vi "SN_parser_new.vi"(6 "Length range":T1, 7 "Parse mode":T4, 8 "error in (no error)":errorcluster, 9 "JSON string":string, 10 "Device Type":T3, 11 "Serial Number in":string) -> (0 "error out":errorcluster, 1 "Device Type out":T2, 2 "SN ok?":bool, 3 "Serial Number out":string)   [LabVIEW 2024]
uses:
  controls/SN_parse_mode.ctl
  controls/SN_device_type.ctl
  controls/SN_device_type_out.ctl
  controls/SN_length.ctl
  libraries/EV QSM support/controls/Data.ctl
  libraries/EV QSM support/support/queue state & data (Array).vi
  <vilib>/Utility/error.llb/Error Cluster From Error Code.vi
  <vilib>/ErrorRing/Error Ring.xnode
  libraries/EV QSM support/Ev Queued SM API.lvlib
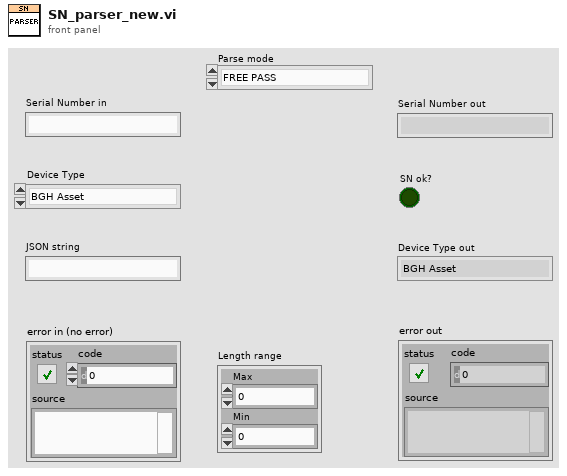
[diagram p1: front panel]
types:
  T1 = typedef "SN_length.ctl" = cluster{"Max":i32, "Min":i32}
  T2 = typedef "SN_device_type_out.ctl" = enum16{"BGH Asset", "BGH Product", "SAMSUNG Product", "GENERIC Product", "No Product", "_"}
  T3 = typedef "SN_device_type.ctl" = enum16{"BGH Asset", "BGH Product", "SAMSUNG Product"}
  T4 = typedef "SN_parse_mode.ctl" = enum16{"FREE PASS", "LENGTH BASED", "REGEX BASED", "AUTO"}
  T5 = typedef "Ev Queued SM API.lvlib/Data.ctl" = cluster{"SN ok?":bool, "SN empty?":bool, "SN":string, "JSON string":string, "Parse mode":T4, "Length range":T1, "Device Type":T3, "Device Type out":T2}
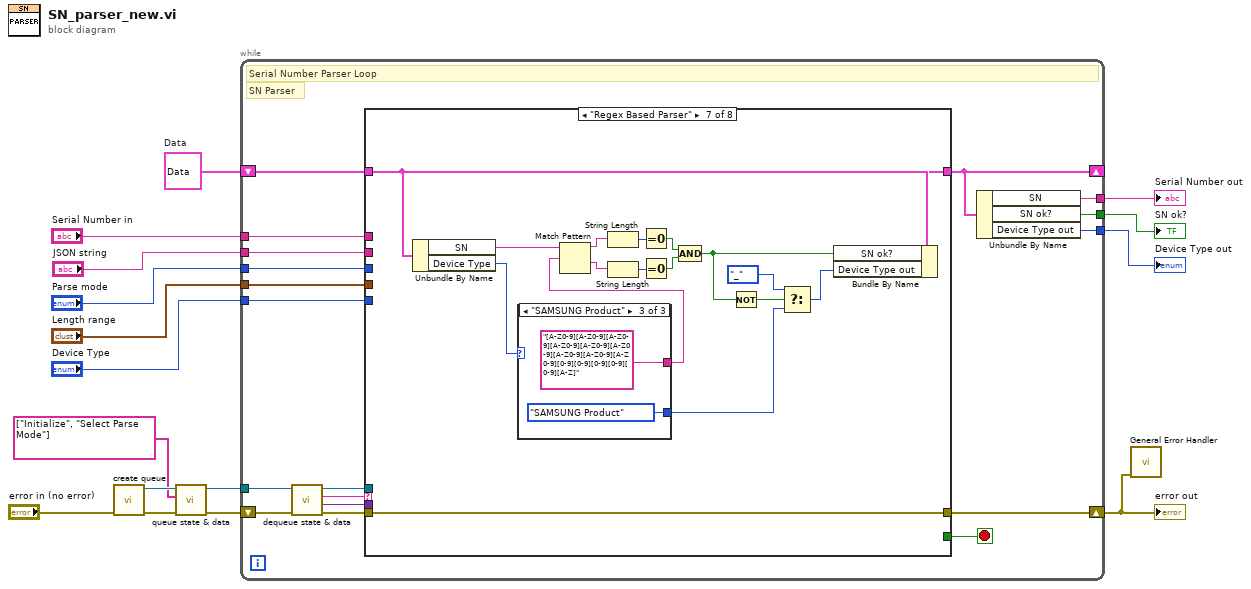
[diagram p0: block diagram]
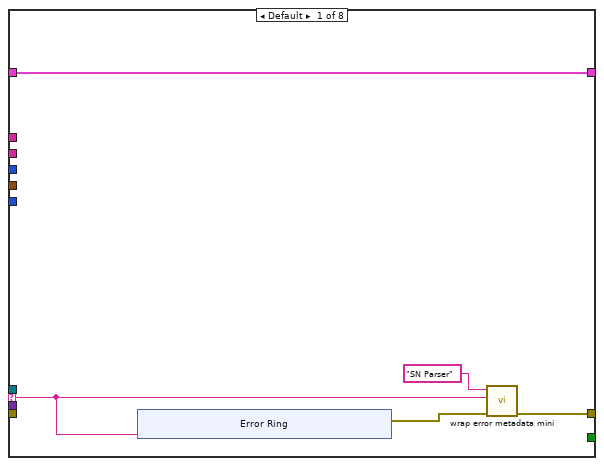
[diagram p2: hidden frame]
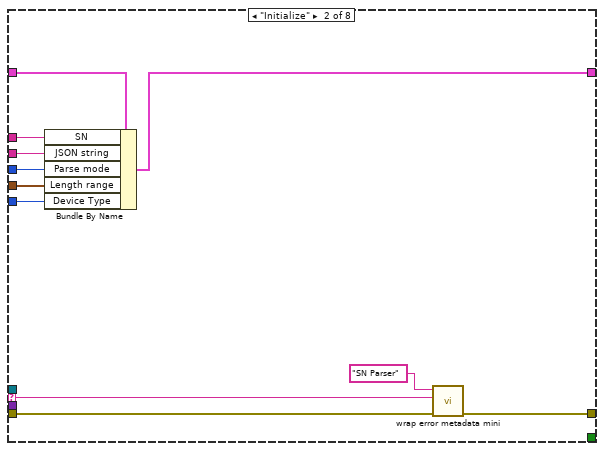
[diagram p3: hidden frame]
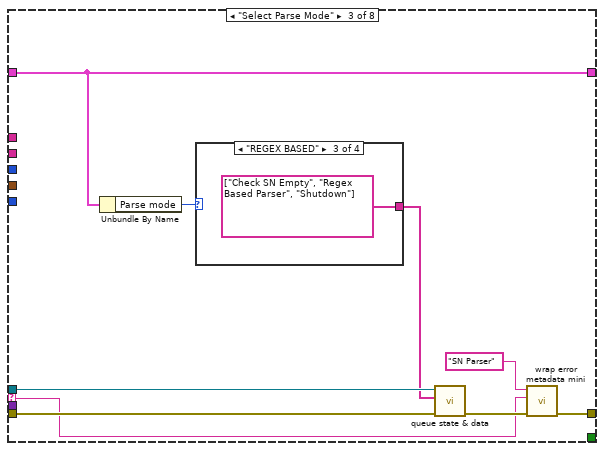
[diagram p4: hidden frame]
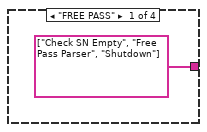
[diagram p5: hidden frame]
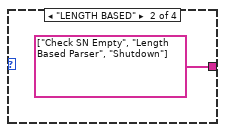
[diagram p6: hidden frame]
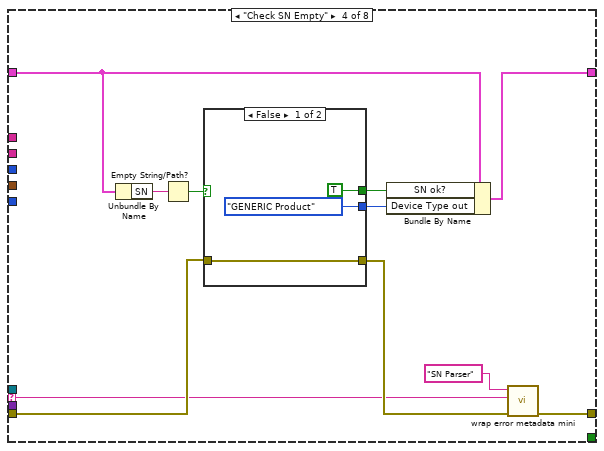
[diagram p8: hidden frame]
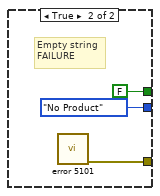
[diagram p9: hidden frame]
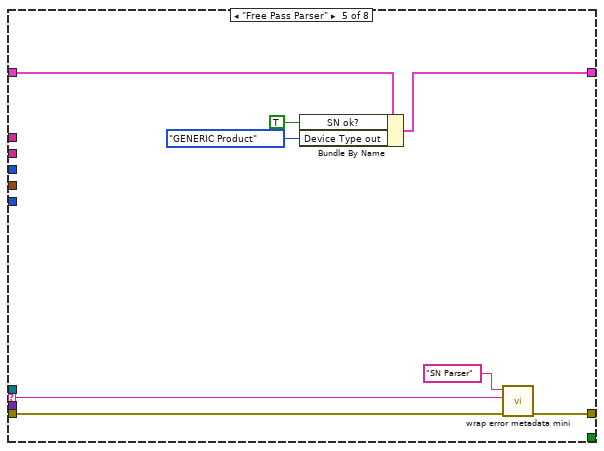
[diagram p10: hidden frame]
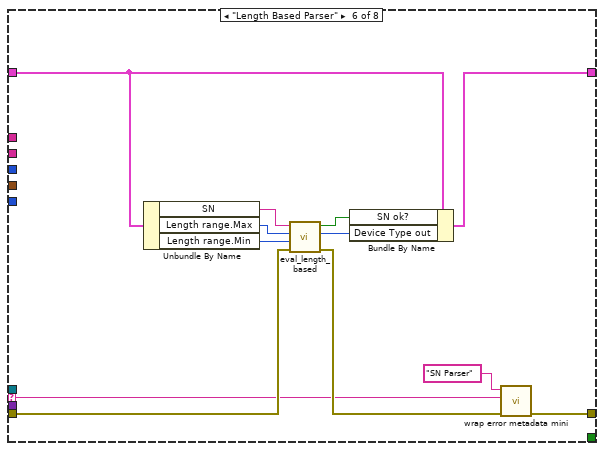
[diagram p11: hidden frame]
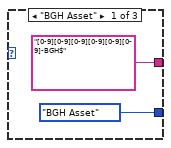
[diagram p12: hidden frame]
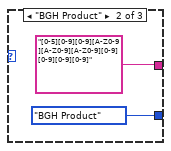
[diagram p13: hidden frame]
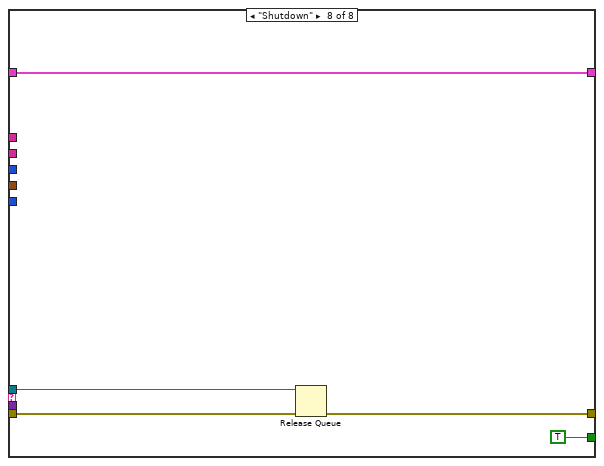
[diagram p14: hidden frame]
diagram:
  w12 = T5 {"SN ok?"=FALSE, "SN empty?"=FALSE, "SN"="", "JSON string"="", "Parse mode"=enum."FREE PASS", "Length range"={"Max"=0, "Min"=0}, "Device Type"=enum."BGH Asset", "Device Type out"=enum."BGH Asset"}  # Data
  n1 = call "create queue.vi"("error in (no error)"="error in (no error)") -> ("error out"=w14:errorcluster, "queue out"=w16:refnum<queue>)  [unwired: 9 in]
  n2 = call-poly "queue state & data.vi"("error in (no error)"=w14, "State Array"=string[] ["Initialize", "Select Parse Mode"], "queue in"=w16) -> ("error out"=w15:errorcluster, "queue out"=w13:refnum<queue>)  [unwired: 7 in]
  n3 = while {
    shift-right: [w17] -> w1
    shift-left: w15 -> [w31]
    tunnel: w13 -> [w29]
    shift-right: [w22] -> _
    shift-left: w12 -> [w28]
    tunnel: "Serial Number in" -> [w27]
    tunnel: "JSON string" -> [w26]
    tunnel: "Parse mode" -> [w25]
    tunnel: "Length range" -> [w24]
    tunnel: "Device Type" -> [w23]
    tunnel: [w19] -> w4
    tunnel: [w21] -> w3
    tunnel: [w20] -> w2
    stop <- w34 stop-if-true
    # "SN Parser"
    # "Serial Number Parser Loop"
    n4 = call "dequeue state & data.vi"("error in (no error)"=w31, "queue in"=w29) -> ("error out"=w33:errorcluster, "State Data"=w32:variant, "State"=w18:string, "queue out"=w30:refnum<queue>)  [unwired: 6 in]
    n5 = case shown="\"Regex Based Parser\"" w18 {
      selector: w18 -> [w35 w49 w58 w70 w90 w95 _ _]
      tunnel: w33 -> [_ w50 w65 w77 w89 w106 w123 w133]
      tunnel: [w36 w48 w59 w71 w91 w96 w123 w131] -> w17
      tunnel: [_ _ _ _ _ _ _ TRUE] -> w34
      tunnel: w30 -> [_ _ w66 _ _ _ _ w132]
      tunnel: w32 -> [_ _ _ _ _ _ _ _]
      tunnel: w28 -> [w39 w57 w63 w80 w94 w102 w113 w130]
      tunnel: [w39 w56 w63 w79 w93 w99 w112 w130] -> w22
      tunnel: w27 -> [_ w55 _ _ _ _ _ _]
      tunnel: w26 -> [_ w54 _ _ _ _ _ _]
      tunnel: w25 -> [_ w52 _ _ _ _ _ _]
      tunnel: w24 -> [_ w53 _ _ _ _ _ _]
      tunnel: w23 -> [_ w47 _ _ _ _ _ _]
      frame Default {
        n6 = xnode ("Error Ring")("parameter 0"=w35) -> ("error out"=w37:errorcluster)
        n7 = call "wrap error metadata mini.vi"("error in (no error)"=w37, "state name"=w35, "task name"="SN Parser") -> ("error out"=w36:errorcluster)  [unwired: 8 in]
      }
      frame "Initialize" {
        n8 = Bundle By Name(cluster=w57, "SN"=w55, "JSON string"=w54, "Parse mode"=w52, "Length range"=w53, "Device Type"=w47) -> (w56:T5)
        n9 = call "wrap error metadata mini.vi"("error in (no error)"=w50, "state name"=w49, "task name"="SN Parser") -> ("error out"=w48:errorcluster)  [unwired: 8 in]
      }
      frame "Select Parse Mode" {
        n10 = Unbundle By Name(w63) -> ("Parse mode"=w62:T4)
        n11 = case shown="\"REGEX BASED\"" w62 {
          tunnel: [string[] ["Check SN Empty", "Free Pass Parser", "Shutdown"] string[] ["Check SN Empty", "Length Based Parser", "Shutdown"] string[] ["Check SN Empty", "Regex Based Parser", "Shutdown"] _] -> w64
          frame "FREE PASS" {
          }
          frame "LENGTH BASED" {
          }
          frame "REGEX BASED" {
          }
          frame "AUTO" {
          }
        }
        n12 = call-poly "queue state & data.vi"("error in (no error)"=w65, "State Array"=w64, "queue in"=w66) -> ("error out"=w60:errorcluster)  [unwired: 7 in, 1 out]
        n13 = call "wrap error metadata mini.vi"("error in (no error)"=w60, "state name"=w58, "task name"="SN Parser") -> ("error out"=w59:errorcluster)  [unwired: 8 in]
      }
      frame "Check SN Empty" {
        n14 = Unbundle By Name(w80) -> ("SN"=w75:string)
        n15 = Empty String/Path?(string/path=w75) -> (empty?=w76:bool)
        n16 = case shown="False" w76 {
          tunnel: [TRUE FALSE] -> w78
          tunnel: [w82 w84] -> w72
          tunnel: w77 -> [w82 _]
          tunnel: [SN_device_type_out."GENERIC Product" ("Device Type out") SN_device_type_out."No Product" ("Device Type out")] -> w74
          frame False {
          }
          frame True {
            # "Empty string\nFAILURE"
            n17 = call "error 5101.vi"() -> ("error out"=w84:errorcluster)  [unwired: 11 in]
          }
        }
        n18 = Bundle By Name(cluster=w80, "SN ok?"=w78, "Device Type out"=w74) -> (w79:T5)
        n19 = call "wrap error metadata mini.vi"("error in (no error)"=w72, "state name"=w70, "task name"="SN Parser") -> ("error out"=w71:errorcluster)  [unwired: 8 in]
      }
      frame "Free Pass Parser" {
        n20 = Bundle By Name(cluster=w94, "SN ok?"=TRUE, "Device Type out"=SN_device_type_out."GENERIC Product") -> (w93:T5)
        n21 = call "wrap error metadata mini.vi"("error in (no error)"=w89, "state name"=w90, "task name"="SN Parser") -> ("error out"=w91:errorcluster)  [unwired: 8 in]
      }
      frame "Length Based Parser" {
        n22 = Unbundle By Name(w102) -> ("SN"=w103:string, "Length range.Max"=w105:i32, "Length range.Min"=w104:i32)
        n23 = call "eval_length_based.vi"("error in (no error)"=w106, "Min"=w104, "Max"=w105, "SN"=w103) -> ("error out"=w97:errorcluster, "Device Type out"=w100:T2, "SN ok?"=w101:bool)  [unwired: 5 in]
        n24 = Bundle By Name(cluster=w102, "SN ok?"=w101, "Device Type out"=w100) -> (w99:T5)
        n25 = call "wrap error metadata mini.vi"("error in (no error)"=w97, "state name"=w95, "task name"="SN Parser") -> ("error out"=w96:errorcluster)  [unwired: 8 in]
      }
      frame "Regex Based Parser" {
        n26 = Unbundle By Name(w113) -> ("SN"=w122:string, "Device Type"=w114:T3)
        n27 = case shown="\"SAMSUNG Product\"" w114 {
          tunnel: ["[0-9][0-9][0-9][0-9][0-9][0-9]-BGH$" "[0-5][0-9][0-9][A-Z0-9][A-Z0-9][A-Z0-9][0-9][0-9][0-9][0-9]" "[A-Z0-9][A-Z0-9][A-Z0-9][A-Z0-9][A-Z0-9][A-Z0-9][A-Z0-9][A-Z0-9][A-Z0-9][0-9][0-9][0-9][0-9][0-9][A-Z]"] -> w115
          tunnel: [SN_device_type_out."BGH Asset" ("Device Type out") SN_device_type_out."BGH Product" ("Device Type out") SN_device_type_out."SAMSUNG Product" ("Device Type out")] -> w111
          frame "BGH Asset" {
          }
          frame "BGH Product" {
          }
          frame "SAMSUNG Product" {
          }
        }
        n28 = Match Pattern(string=w122, regular expression=w115) -> (before substring=w116:string, after substring=w117:string)  [unwired: 1 in, 2 out]
        n29 = String Length(string=w116) -> (length=w118:i32)
        n30 = String Length(string=w117) -> (length=w119:i32)
        n31 = Equal To 0?(x=w118) -> (x = 0?=w121:bool)
        n32 = Equal To 0?(x=w119) -> (x = 0?=w120:bool)
        n33 = Compound Arithmetic op=AND(w121, w120) -> (w107:bool)
        n34 = Not(x=w107) -> (.not. x?=w108:bool)
        n35 = Select(t=SN_device_type_out."_", s=w108, f=w111) -> (s? t:f=w110:T2)
        n36 = Bundle By Name(cluster=w113, "SN ok?"=w107, "Device Type out"=w110) -> (w112:T5)
      }
      frame "Shutdown" {
        n37 = Release Queue(queue=w132, error in (no error)=w133) -> (error out=w131:errorcluster)  [unwired: 1 in, 2 out]
      }
    }
    n38 = Unbundle By Name(w22) -> ("SN"=w21:string, "SN ok?"=w20:bool, "Device Type out"=w19:T2)
  }
  "error out" <- w1
  "SN ok?" <- w2
  "Device Type out" <- w4
  "Serial Number out" <- w3
  n39 = call <vilib>:"General Error Handler.vi"("error in (no error)"=w1) -> ()  [unwired: 10 in, 5 out]
